vi "Post-Build Action.vi"(4 "measurement plugin service":refnum<class "Measurement Plugin Service.lvclass">, 5 "files generated by build":path[](array[path]), 6 "top level/always included VIs":path[](array[path]), 7 "destination path":path, 8 "error in":errorcluster, 9 "target name":string, 10 "build specification name":string, 11 "project path":path) -> (0 "error out":errorcluster)   [LabVIEW 2021, in "NI Measurement Plug-In SDK.lvlib"]
uses:
  NI Measurement Plug-In SDK.lvlib
  <vilib>/Utility/config.llb/NI_LVConfig.lvlib
  <vilib>/Utility/config.llb/Write Key (String).vi
  Measurement Plugin Service/Measurement Plugin Service.lvclass
  Users/peter/OneDrive - Emerson/Desktop/VI Info/VI Info.lvlib
  <vilib>/JDP Science/JDP Science Common Utilities/Base64/Base64 Support.lvlib
  e44bdc69-f632-4107-b999-8ee91106dd9d.vi
  <vilib>/wsapi/NI_WebServices.lvlib
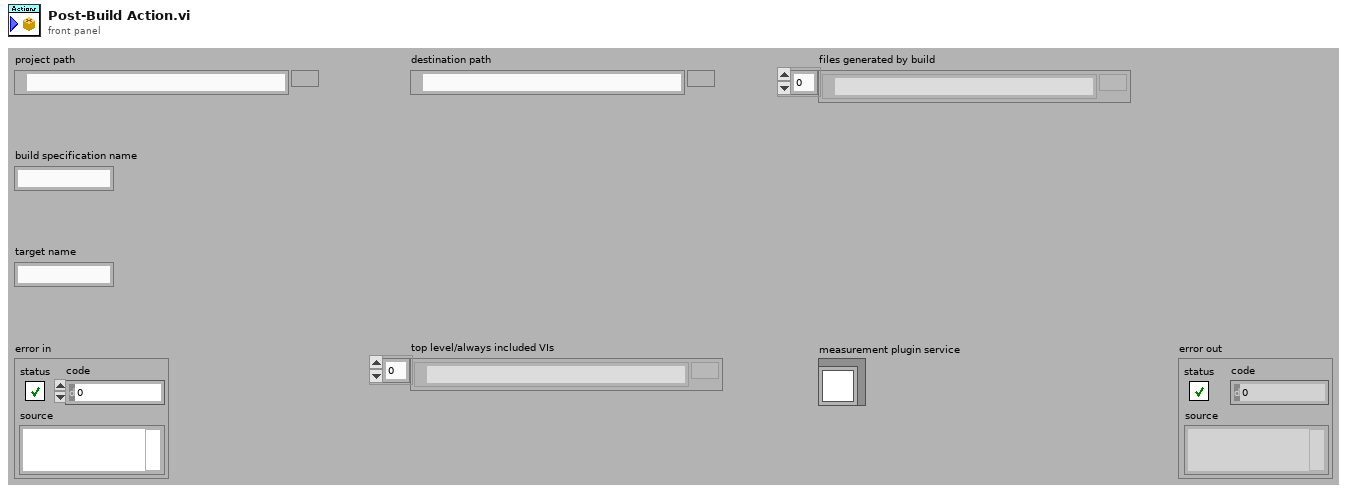
[diagram p1: front panel]
types:
  T1 = cluster{"target name":string, "top level/always included VIs":path[], "project path":path, "destination path":path, "build specification name":string, "files generated by build":path[]}
  T2 = typedef "NI Measurement Plug-In SDK.lvlib/User Interface Details.ctl" = cluster{"file url":string}
  T3 = typedef "NI Measurement Plug-In SDK.lvlib/Service Descriptor.ctl" = cluster{"measurement details":T4, "description URL":string, "service class":string, "measurement annotations":T5[]}
  T4 = typedef "NI Measurement Plug-In SDK.lvlib/Measurement Details.ctl" = cluster{"display name":string, "version":string}
  T5 = typedef "NI Measurement Plug-In SDK.lvlib/Measurement Annotation.ctl" = cluster{"key":string, "value":string}
  T6 = typedef "NI Measurement Plug-In SDK.lvlib/Measurement Plugin Service.lvclass/Plugin Paths.ctl" = cluster{"get service descriptor VI path":path, "get type specializations VI path":path, "get UI details VI path":path, "measurement logic VI path":path, "measurement configuration ctl path":path, "measurement results ctl path":path}
  T7 = typedef "imagedata.ctl" = cluster{"image type":i32, "image depth":i32, "image":u8[], "mask":u8[], "colors":u32[], "Rectangle":cluster{"left":i16, "top":i16, "right":i16, "bottom":i16}}
  T8 = cluster{"Documentation/Icon":cluster{"Name":string, "Description":string, "ImageData":T7}, "Images":T7[]}
  T9 = typedef "NI_LVConfig.lvlib/Config Data RefNum.ctl" = refnum<k1>
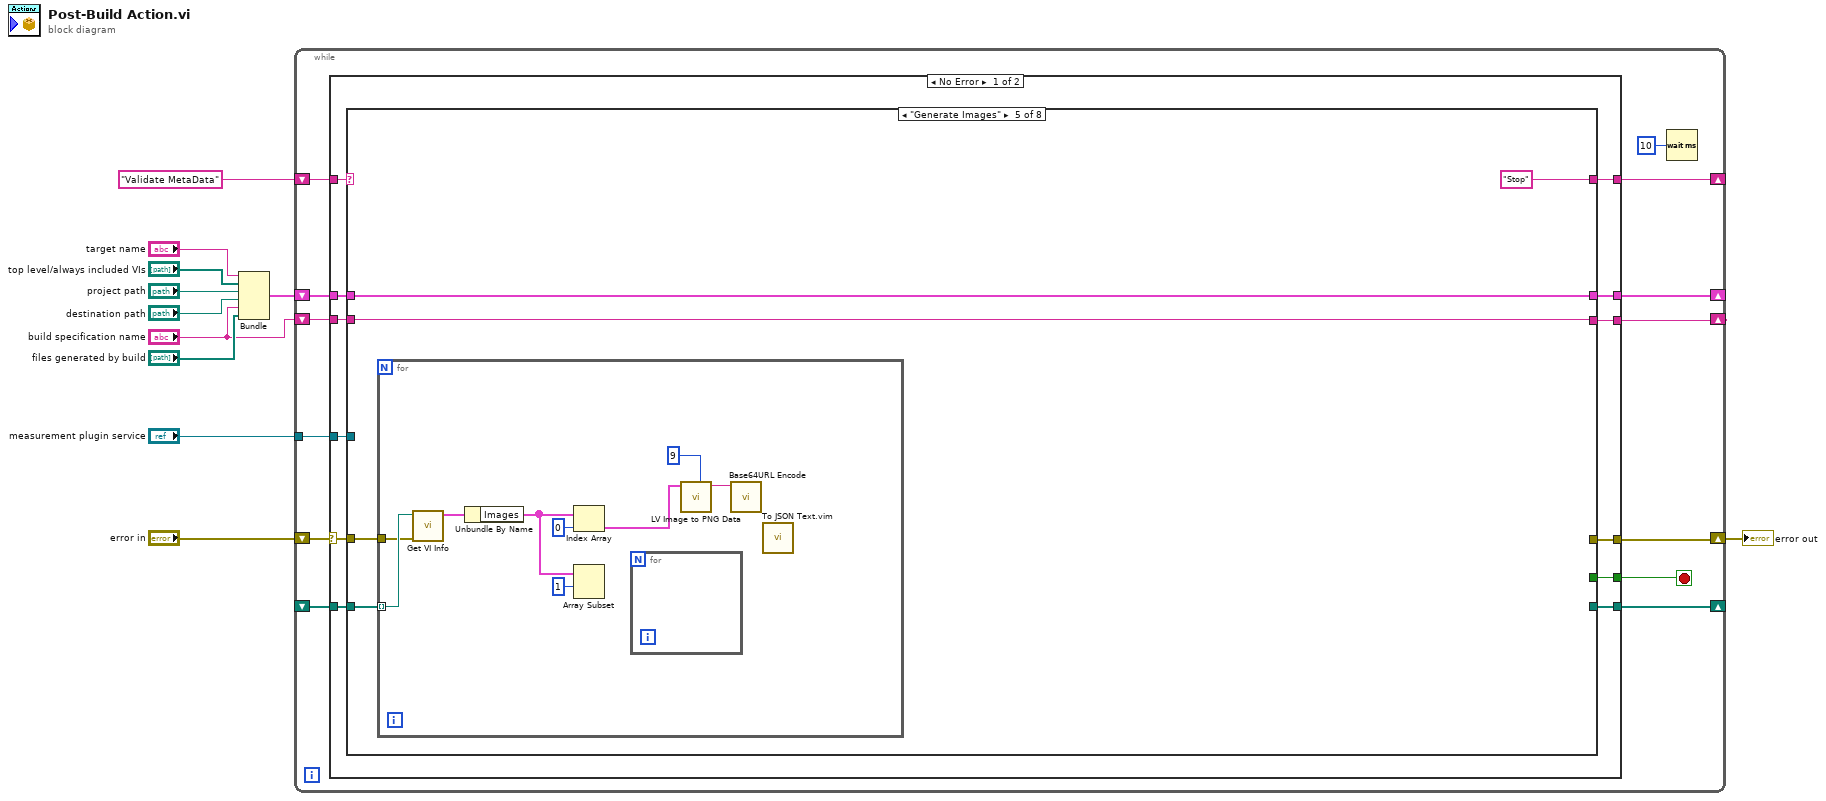
[diagram p0: block diagram]
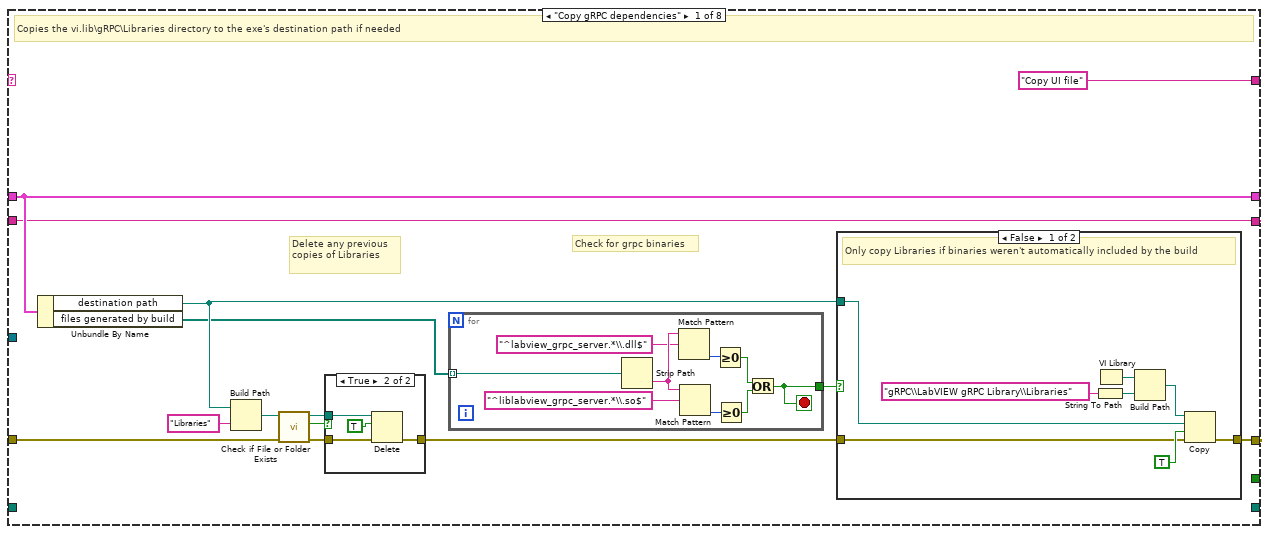
[diagram p2: hidden frame]
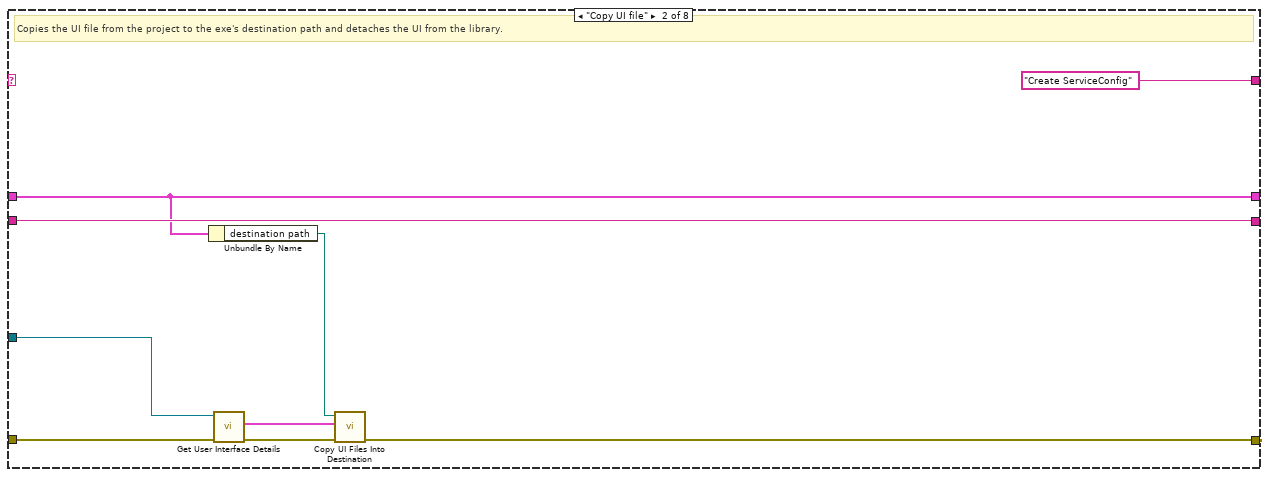
[diagram p5: hidden frame]
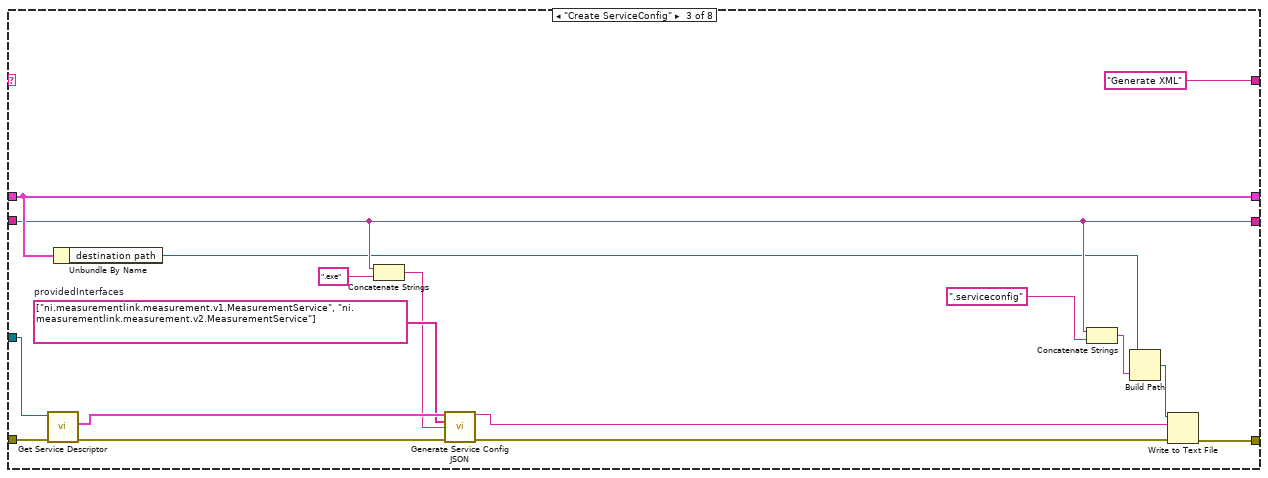
[diagram p6: hidden frame]
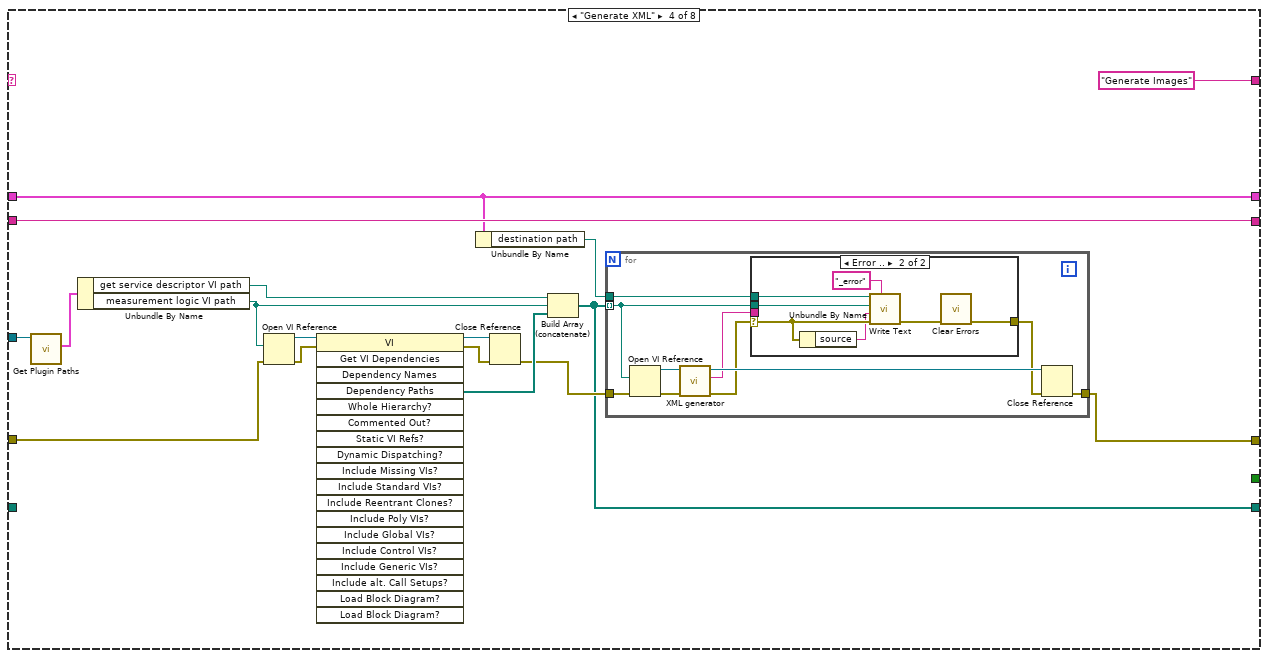
[diagram p7: hidden frame]
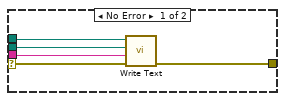
[diagram p8: hidden frame]
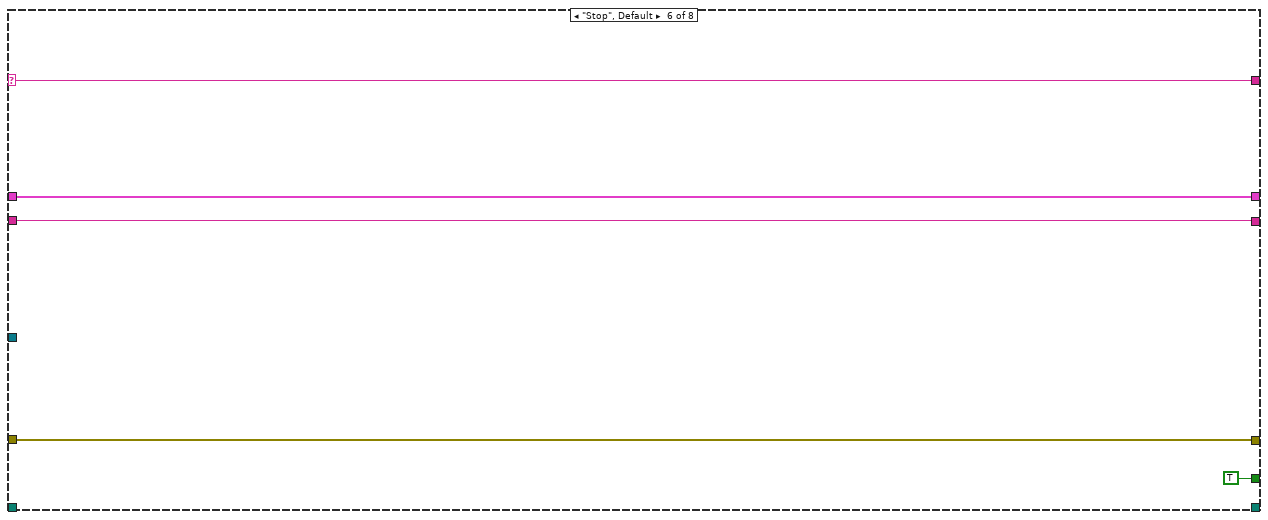
[diagram p9: hidden frame]
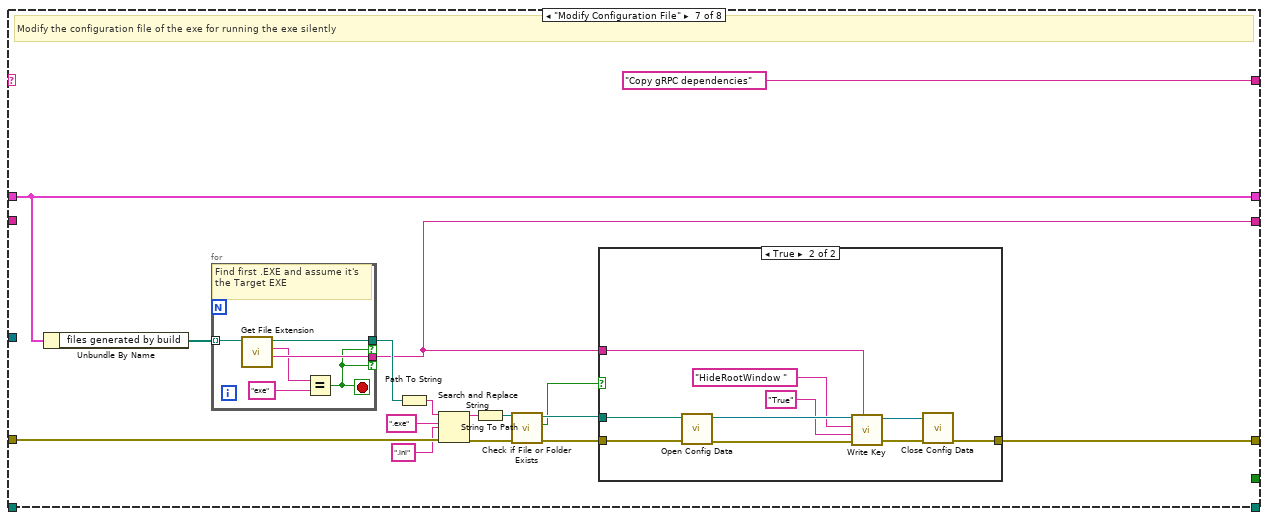
[diagram p10: hidden frame]
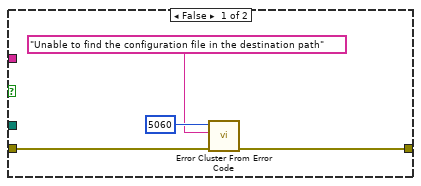
[diagram p11: hidden frame]
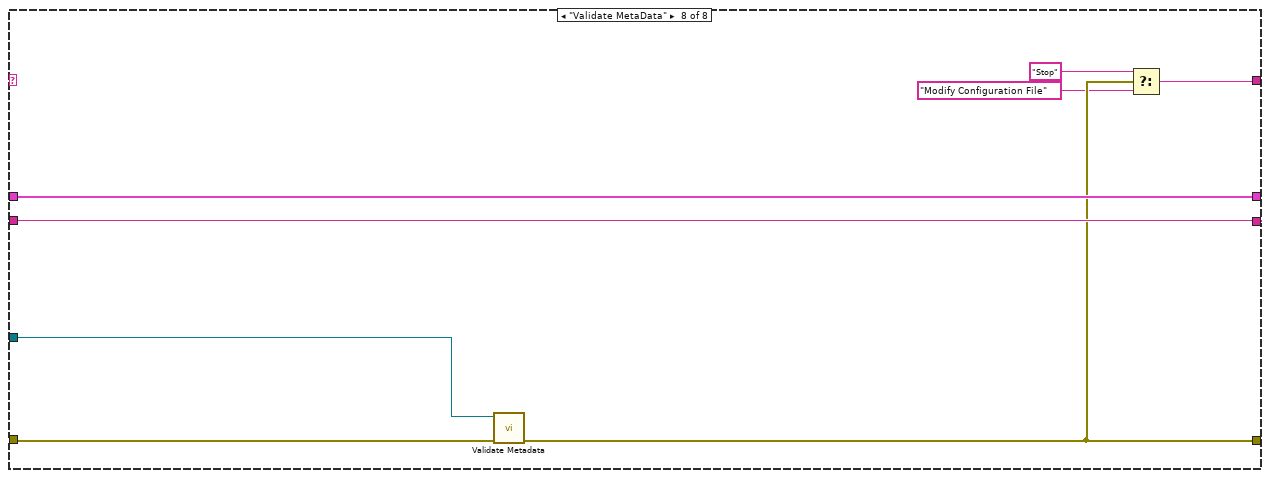
[diagram p12: hidden frame]
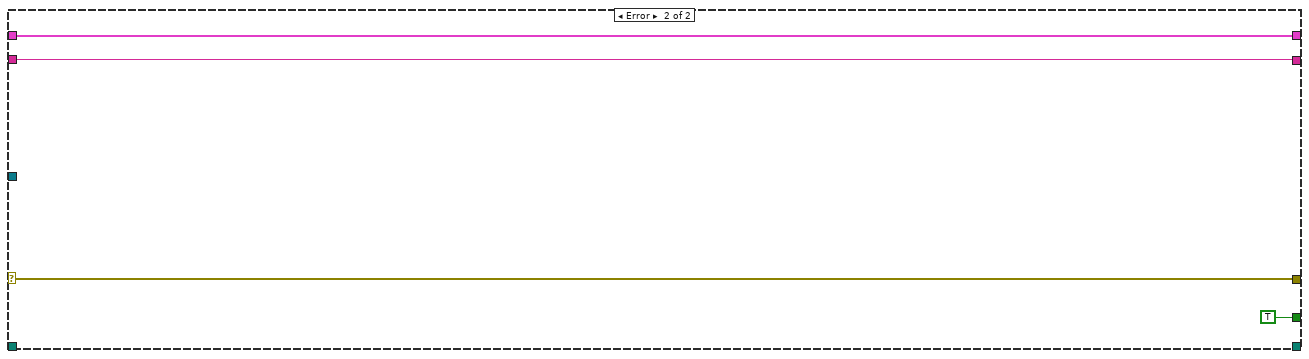
[diagram p13: hidden frame]
diagram:
  n1 = Bundle("target name"="target name", "top level/always included VIs"="top level/always included VIs", "project path"="project path", "destination path"="destination path", "build specification name"="build specification name", "files generated by build"="files generated by build") -> (w5:T1)  [unwired: 1 in]
  n2 = while {
    shift-right: [w21] -> _
    shift-left: w5 -> [w22]
    shift-right: [w20] -> w3
    shift-left: "error in" -> [w17]
    shift-right: [w19] -> _
    shift-left: "Validate MetaData" -> [w23]
    shift-right: [w16] -> _
    shift-left: "build specification name" -> [w15]
    tunnel: "measurement plugin service" -> [w14]
    shift-right: [w13] -> _
    shift-left: _ -> [w12]
    stop <- w18 stop-if-true
    n3 = case shown="No Error" w17 {
      selector: w17 -> [w30 w204]
      tunnel: w23 -> [w36 _]
      tunnel: w22 -> [w35 w205]
      tunnel: [w34 w205] -> w21
      tunnel: [w33 w204] -> w20
      tunnel: [w32 _] -> w19
      tunnel: [w31 TRUE] -> w18
      tunnel: [w29 w202] -> w16
      tunnel: w15 -> [w28 w202]
      tunnel: w14 -> [w27 _]
      tunnel: [w26 _] -> w13
      tunnel: w12 -> [w25 _]
      frame No Error {
        n4 = case shown="\"Generate Images\"" w36 {
          selector: w36 -> [_ _ _ _ _ w155 _ _]
          tunnel: w35 -> [w48 w79 w99 w114 w143 w157 w169 w201]
          tunnel: [w48 w79 w99 w114 w143 w157 w169 w201] -> w34
          tunnel: w30 -> [w40 w77 w89 w105 w139 w154 w167 w199]
          tunnel: [w50 w78 w92 w103 _ w154 w173 w197] -> w33
          tunnel: ["Copy UI file" "Create ServiceConfig" "Generate XML" "Generate Images" "Stop" w155 "Copy gRPC dependencies" w194] -> w32
          tunnel: [_ _ _ _ _ TRUE _ _] -> w31
          tunnel: [w47 w81 w96 w116 w142 w153 w159 w200] -> w29
          tunnel: w28 -> [w47 w81 w96 w116 w142 w153 _ w200]
          tunnel: w27 -> [_ w75 w90 w113 _ _ _ w198]
          tunnel: [_ _ _ w100 _ _ _ _] -> w26
          tunnel: w25 -> [_ _ _ _ w140 _ _ _]
          frame "Copy gRPC dependencies" {
            # "Delete any previous copies of Libraries"
            # "Check for grpc binaries"
            # "Copies the vi.lib\\gRPC\\Libraries directory to the exe's destination path if needed"
            n5 = Unbundle By Name(w48) -> ("destination path"=w39:path, "files generated by build"=w37:path[])
            n6 = Build Path(base path=w39, name or relative path="Libraries") -> (appended path=w45:path)
            n7 = call <vilib>:"Check if File or Folder Exists.vi"("error in (no error)"=w40, "path"=w45) -> ("error out"=w44:errorcluster, "file or folder exists?"=w42:bool, "dup path"=w43:path)  [unwired: 7 in]
            n8 = case shown="True" w42 {
              tunnel: w44 -> [w60 w64]
              tunnel: [w60 w63] -> w38
              tunnel: w43 -> [_ w61]
              frame False {
              }
              frame True {
                n9 = Delete(path (use dialog)=w61, entire hierarchy (F)=TRUE ("confirm (F)"), error in=w64) -> (error out=w63:errorcluster)  [unwired: 2 in, 2 out]
              }
            }
            n10 = for {
              tunnel: [w51] -> w46
              tunnel: w37 -> [w56] mode=indexing
              stop <- w51 stop-if-true
              n11 = Strip Path(path=w56) -> (name=w59:string)  [unwired: 1 out]
              n12 = Match Pattern(string=w59, regular expression="^labview_grpc_server.*\\.dll$" ("pattern")) -> (offset past match=w55:i32)  [unwired: 1 in, 3 out]
              n13 = Match Pattern(string=w59, regular expression="^liblabview_grpc_server.*\\.so$" ("pattern")) -> (offset past match=w54:i32)  [unwired: 1 in, 3 out]
              n14 = Greater Or Equal To 0?(x=w55) -> (x >= 0?=w53:bool)
              n15 = Greater Or Equal To 0?(x=w54) -> (x >= 0?=w52:bool)
              n16 = Or(x=w53, y=w52) -> (x .or. y?=w51:bool)
            }
            n17 = case shown="False" w46 {
              tunnel: [w68 w73] -> w50
              tunnel: w39 -> [w66 _]
              tunnel: w38 -> [w65 w73]
              frame False {
                # "Only copy Libraries if binaries weren't automatically included by the build"
                n18 = String To Path(string="gRPC\\LabVIEW gRPC Library\\Libraries") -> (path=w70:path)
                n19 = VI Library() -> (path=w72:path)
                n20 = Build Path(base path=w72, name or relative path=w70) -> (appended path=w69:path)
                n21 = Copy(8:w65, 9:TRUE ("overwrite (F)"), 10:w66, 11:w69) -> (0:w68:errorcluster)  [unwired: 1 in, 2 out]
              }
              frame True {
              }
            }
          }
          frame "Copy UI file" {
            # "Copies the UI file from the project to the exe's destination path and detaches the UI from the library."
            n22 = Unbundle By Name(w79) -> ("destination path"=w80:path)
            n23 = call-dynamic "Get User Interface Details.vi"("error in"=w77, "measurement plugin service in"=w75) -> ("error out"=w76:errorcluster, "user interface details"=w74:T2[])  [unwired: 7 in, 1 out]
            n24 = call "Copy UI Files Into Destination.vi"("error in"=w76, "user interface details"=w74, "destination path"=w80) -> ("error out"=w78:errorcluster)  [unwired: 8 in]
          }
          frame "Create ServiceConfig" {
            w84 = string[] ["ni.measurementlink.measurement.v1.MeasurementService", "ni.measurementlink.measurement.v2.MeasurementService"]  # providedInterfaces
            n25 = call "Get Service Descriptor.vi"("error in"=w89, "measurement plugin service in"=w90) -> ("error out"=w88:errorcluster, "service descriptor"=w85:T3)  [unwired: 7 in, 1 out]
            n26 = Unbundle By Name(w99) -> ("destination path"=w94:path)
            n27 = Concatenate Strings(w96, ".exe" ("string")) -> (w83:string)
            n28 = call "Generate Service Config JSON.vi"("service descriptor"=w85, "provided interfaces"=w84, "path"=w83, "error in"=w88) -> ("service config JSON"=w86:string, "error out"=w87:errorcluster)  [unwired: 10 in]
            n29 = Concatenate Strings(w96, ".serviceconfig" ("string")) -> (w93:string)
            n30 = Build Path(base path=w94, name or relative path=w93) -> (appended path=w91:path)
            n31 = Write to Text File(file (use dialog)=w91, text=w86, error in=w87) -> (error out=w92:errorcluster)  [unwired: 1 in, 2 out]
          }
          frame "Generate XML" {
            n32 = call-dynamic "Get Plugin Paths.vi"("measurement plugin service in"=w113) -> ("plugin paths"=w112:T6)  [unwired: 8 in, 2 out]
            n33 = Unbundle By Name(w112) -> ("get service descriptor VI path"=w102:path, "measurement logic VI path"=w109:path)
            n34 = Open VI Reference(vi path=w109, error in (no error)=w105) -> (vi reference=w111:refnum<vi>, error out=w106:errorcluster)  [unwired: 4 in]
            n35 = invoke class="VI" method="Get VI Dependencies"(reference=w111, error in=w106) -> (reference out=w108:refnum<vi>, error out=w107:errorcluster, "Dependency Paths"=w110:path[])  [unwired: 17 in, 16 out]
            n36 = Unbundle By Name(w114) -> ("destination path"=w101:path)
            n37 = Close Reference(reference=w108, error in (no error)=w107) -> (error out=w104:errorcluster)
            n38 = Build Array (concatenate)(w102, w109, w110) -> (w100:path[])
            n39 = for {
              tunnel: w100 -> [w120] mode=indexing
              tunnel: w104 -> [w124]
              tunnel: [w123] -> w103
              tunnel: w101 -> [w117]
              n40 = Open VI Reference(vi path=w120, error in (no error)=w124) -> (vi reference=w126:refnum<vi>, error out=w125:errorcluster)  [unwired: 4 in]
              n41 = call "XML generator.vi"("error in (no error)"=w125, "vi"=w126) -> ("error out"=w118:errorcluster, "XML"=w119:string, "vi out"=w122:refnum<vi>)  [unwired: 7 in]
              n42 = case shown="Error .." w118 {
                selector: w118 -> [w131 w138]
                tunnel: [w130 w133] -> w121
                tunnel: w120 -> [w129 w135]
                tunnel: w119 -> [w128 _]
                tunnel: w117 -> [w127 w132]
                frame No Error {
                  n43 = call "Write Text.vi"("error in (no error)"=w131, "Content"=w128, "VI Path in"=w129, "Directory Path in"=w127) -> ("error out"=w130:errorcluster)  [unwired: 5 in, 2 out]
                }
                frame Error {
                  n44 = Unbundle By Name(w138) -> ("source"=w137:string)
                  n45 = call "Write Text.vi"("Filename Suffix"="_error", "error in (no error)"=w138, "Content"=w137, "VI Path in"=w135, "Directory Path in"=w132) -> ("error out"=w134:errorcluster)  [unwired: 4 in, 2 out]
                  n46 = call <vilib>:"Clear Errors.vi"("error in (no error)"=w134) -> ("error out"=w133:errorcluster)  [unwired: 5 in, 1 out]
                }
              }
              n47 = Close Reference(reference=w122, error in (no error)=w121) -> (error out=w123:errorcluster)
            }
          }
          frame "Generate Images" {
            n48 = for {
              tunnel: w140 -> [w152] mode=indexing
              tunnel: w139 -> [w151]
              n49 = call "Get VI Info.vi"("error in (no error)"=w151, "VI Path in"=w152) -> ("VI Info out"=w150:T8)  [unwired: 8 in, 1 out]
              n50 = Unbundle By Name(w150) -> ("Images"=w148:T7[])
              n51 = Index Array(array=w148, index=0) -> (element=w146:T7)
              n52 = Array Subset(array=w148, index=1) -> ()  [unwired: 1 in, 1 out]
              n53 = for {
              }
              n54 = call <vilib>:"LV Image to PNG Data.vi"("compression (none)"=9, "image data"=w146) -> ("png data"=w144:string)  [unwired: 8 in, 1 out]
              n55 = call <vilib>:"Base64URL Encode.vi"("String to Encode"=w144) -> ()  [unwired: 10 in, 1 out]
              n56 = call "To JSON Text.vim"() -> ()  [unwired: 10 in, 2 out]
            }
          }
          frame "Stop", Default {
          }
          frame "Modify Configuration File" {
            # "Modify the configuration file of the exe for running the exe silently"
            n57 = Unbundle By Name(w169) -> ("files generated by build"=w168:path[])
            n58 = for {
              tunnel: w168 -> [w179] mode=indexing
              tunnel: [w178] -> w159 if=w174
              tunnel: [w177] -> w161 if=w174
              stop <- w174 stop-if-true
              # "Find first .EXE and assume it's the Target EXE"
              n59 = call <vilib>:"Get File Extension.vi"("file"=w179) -> ("filename without extension"=w178:string, "lowercase file extension"=w175:string, "dup file"=w177:path)  [unwired: 6 in, 2 out]
              n60 = Equal?(x=w175, y="exe") -> (x = y?=w174:bool)
            }
            n61 = Path To String(path=w161) -> (string=w160:string)
            n62 = Search and Replace String(input string=w160, search string=".exe", replace string=".ini", error in=w167) -> (result string=w164:string, error out=w166:errorcluster)  [unwired: 4 in, 2 out]
            n63 = String To Path(string=w164) -> (path=w163:path)
            n64 = call <vilib>:"Check if File or Folder Exists.vi"("error in (no error)"=w166, "path"=w163) -> ("error out"=w172:errorcluster, "file or folder exists?"=w170:bool, "dup path"=w171:path)  [unwired: 7 in]
            n65 = case shown="True" w170 {
              tunnel: [w182 w193] -> w173
              tunnel: w171 -> [_ w186]
              tunnel: w172 -> [w183 w185]
              tunnel: w159 -> [_ w184]
              frame False {
                n66 = call <vilib>:"Error Cluster From Error Code.vi"("error in (no error)"=w183, "error message (\"\")"="Unable to find the configuration file in the destination path" ("source"), "error code (0)"=5060) -> ("error out"=w182:errorcluster)  [unwired: 6 in]
              }
              frame True {
                n67 = call <vilib>:"Open Config Data.vi"("error in (no error)"=w185, "configuration file path"=w186) -> ("error out"=w192:errorcluster, "refnum"=w191:T9)  [unwired: 7 in, 1 out]
                n68 = call-poly <vilib>:"Write Key.vi"("section"=w184, "error in (no error)"=w192, "value"="True", "key"="HideRootWindow ", "refnum"=w191) -> ("error out"=w189:errorcluster, "refnum out"=w188:T9)  [unwired: 4 in, 1 out]
                n69 = call <vilib>:"Close Config Data.vi"("error in (no error)"=w189, "refnum"=w188) -> ("error out"=w193:errorcluster)  [unwired: 8 in, 1 out]
              }
            }
          }
          frame "Validate MetaData" {
            n70 = call "Validate Metadata.vi"("error in"=w199, "measurement plugin service in"=w198) -> ("error out"=w197:errorcluster)  [unwired: 8 in, 1 out]
            n71 = Select(t="Stop", s=w197, f="Modify Configuration File") -> (s? t:f=w194:string)
          }
        }
      }
      frame Error {
      }
    }
    n72 = Wait (ms)(milliseconds to wait=u32 10 ("millisecond timer value")) -> ()  [unwired: 1 out]
  }
  "error out" <- w3
